vi "8 Bits Write.vi"(6 "E?E1:E2 (E1)":bool=TRUE, 9 "RS":bool, 10 "LCD data/cmd":u8 format="%.0x", 11 "device connection map":T1={"RS"="RS", "R/W"="RW", "E1"="E1", "E2"="E1", "DB0"="DB0", "DB1"="DB1", "DB2"="DB2", "DB3"="DB3", "DB4"="DB4", "DB5"="DB5", "DB6"="DB6", "DB7"="DB7"}) -> ()   [LabVIEW 2017, in "HD44780 FPGA.lvlib"]
uses:
  HD44780 FPGA.lvlib
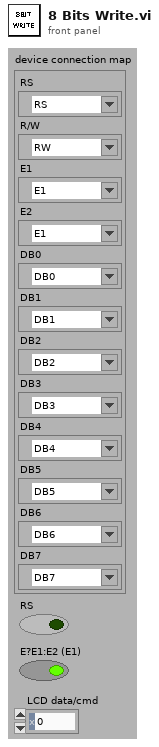
[diagram p1: front panel]
types:
  T1 = cluster{"RS":refnum<k21>, "R/W":refnum<k21>, "E1":refnum<k21>, "E2":refnum<k21>, "DB0":refnum<k21>, "DB1":refnum<k21>, "DB2":refnum<k21>, "DB3":refnum<k21>, "DB4":refnum<k21>, "DB5":refnum<k21>, "DB6":refnum<k21>, "DB7":refnum<k21>}
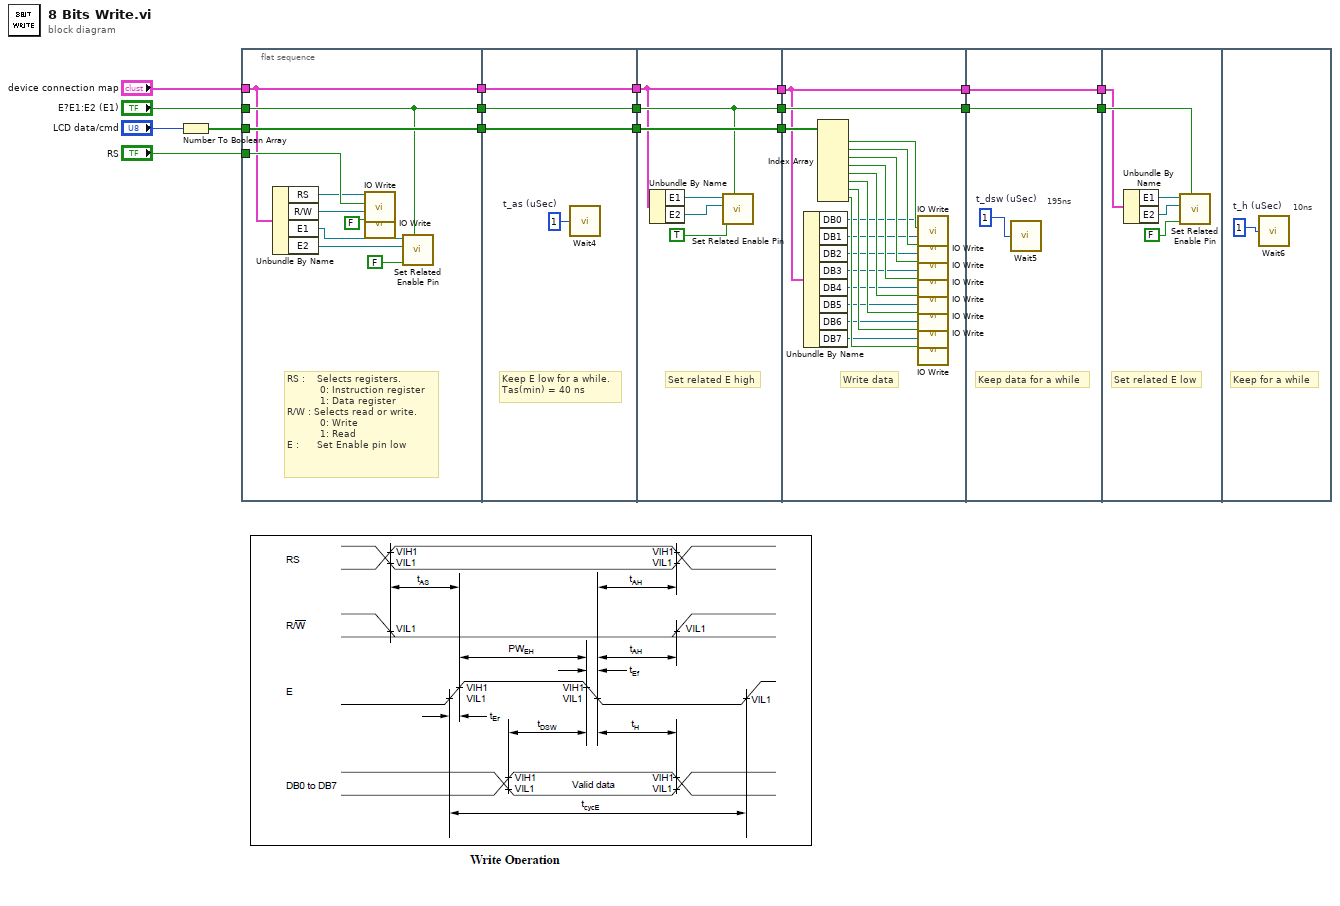
[diagram p0: block diagram]
diagram:
  n1 = Number To Boolean Array(number="LCD data/cmd") -> (Boolean array=w15:bool[])
  n2 = flat-sequence {
    tunnel: [w25] -> w14
    tunnel: [w24] -> w10
    tunnel: [w19] -> w5
    tunnel: "RS" -> [w26]
    tunnel: "E?E1:E2 (E1)" -> [w24]
    tunnel: w15 -> [w25]
    tunnel: "device connection map" -> [w19]
    tunnel: w14 -> [w31]
    tunnel: [w31] -> w13
    tunnel: [w30] -> w11
    tunnel: w10 -> [w30]
    tunnel: [w29] -> w6
    tunnel: w5 -> [w29]
    tunnel: w13 -> [w37]
    tunnel: [w37] -> w12
    tunnel: w11 -> [w36]
    tunnel: [w36] -> w7
    tunnel: w6 -> [w33]
    tunnel: [w33] -> w4
    tunnel: w12 -> [w49]
    tunnel: [w48] -> w8
    tunnel: w7 -> [w48]
    tunnel: w4 -> [w47]
    tunnel: [w47] -> w3
    tunnel: [w59] -> w9
    tunnel: w8 -> [w59]
    tunnel: w3 -> [w58]
    tunnel: [w58] -> w2
    tunnel: w9 -> [w64]
    tunnel: w2 -> [w63]
    frame #0 {
      # "RS :    Selects registers.\n           0: Instruction register  \n           1: Data register\nR/W : Selects read or write.\n           0: Write\n           1: Read\nE :      Set Enable pin low"
      n3 = Unbundle By Name(w19) -> ("RS"=w23:refnum<k21>, "R/W"=w22:refnum<k21>, "E1"=w21:refnum<k21>, "E2"=w20:refnum<k21>)
      n4 = call "IO Write.vi"("data"=w26, "I/O"=w23) -> ()  [unwired: 10 in]
      n5 = call "IO Write.vi"("data"=FALSE, "I/O"=w22) -> ()  [unwired: 10 in]
      n6 = call "Set Related Enable Pin.vi"("E?E1:E2"=w24, "data"=FALSE, "E2"=w20, "E1"=w21) -> ()  [unwired: 8 in]
    }
    frame #1 {
      w32 = u32 1  # t_as (uSec)
      # "Keep E low for a while.\nTas(min) = 40 ns"
      n7 = call "Wait4"("Count(uSec)"=w32) -> ()  [unwired: 1 out]
    }
    frame #2 {
      # "Set related E high"
      n8 = Unbundle By Name(w33) -> ("E1"=w35:refnum<k21>, "E2"=w34:refnum<k21>)
      n9 = call "Set Related Enable Pin.vi"("E?E1:E2"=w36, "data"=TRUE, "E2"=w34, "E1"=w35) -> ()  [unwired: 8 in]
    }
    frame #3 {
      # "Write data"
      n10 = Unbundle By Name(w47) -> ("DB0"=w46:refnum<k21>, "DB1"=w45:refnum<k21>, "DB2"=w44:refnum<k21>, "DB3"=w43:refnum<k21>, "DB4"=w42:refnum<k21>, "DB5"=w41:refnum<k21>, "DB6"=w40:refnum<k21>, "DB7"=w39:refnum<k21>)
      n11 = Index Array(array=w49) -> (element #1=w57:bool, element #2=w56:bool, element #3=w55:bool, element #4=w54:bool, element #5=w53:bool, element #6=w52:bool, element #7=w51:bool, element #8=w50:bool)  [unwired: 8 in]
      n12 = call "IO Write.vi"("data"=w57, "I/O"=w46) -> ()  [unwired: 10 in]
      n13 = call "IO Write.vi"("data"=w56, "I/O"=w45) -> ()  [unwired: 10 in]
      n14 = call "IO Write.vi"("data"=w55, "I/O"=w44) -> ()  [unwired: 10 in]
      n15 = call "IO Write.vi"("data"=w54, "I/O"=w43) -> ()  [unwired: 10 in]
      n16 = call "IO Write.vi"("data"=w53, "I/O"=w42) -> ()  [unwired: 10 in]
      n17 = call "IO Write.vi"("data"=w52, "I/O"=w41) -> ()  [unwired: 10 in]
      n18 = call "IO Write.vi"("data"=w51, "I/O"=w40) -> ()  [unwired: 10 in]
      n19 = call "IO Write.vi"("data"=w50, "I/O"=w39) -> ()  [unwired: 10 in]
    }
    frame #4 {
      w60 = u32 1  # t_dsw (uSec)
      # "Keep data for a while"
      # "195ns"
      n20 = call "Wait5"("Count(uSec)"=w60) -> ()  [unwired: 1 out]
    }
    frame #5 {
      # "Set related E low"
      n21 = Unbundle By Name(w63) -> ("E1"=w62:refnum<k21>, "E2"=w61:refnum<k21>)
      n22 = call "Set Related Enable Pin.vi"("E?E1:E2"=w64, "data"=FALSE, "E2"=w61, "E1"=w62) -> ()  [unwired: 8 in]
    }
    frame #6 {
      w66 = u32 1  # t_h (uSec)
      # "Keep for a while"
      # "10ns"
      n23 = call "Wait6"("Count(uSec)"=w66) -> ()  [unwired: 1 out]
    }
  }
